vi "change_name.vi"(8 "error in (no error)":errorcluster, 9 "SerialNum":string, 10 "New Dev Name":string, 11 "Resources in":refnum<k20>[](array[refnum])) -> (0 "error out":errorcluster, 3 "Changed?":bool)   [LabVIEW 2015]
uses:
  <resource>/objmgr/nisysapi.rc
  <vilib>/nisyscfg/nisyscfg.lvlib
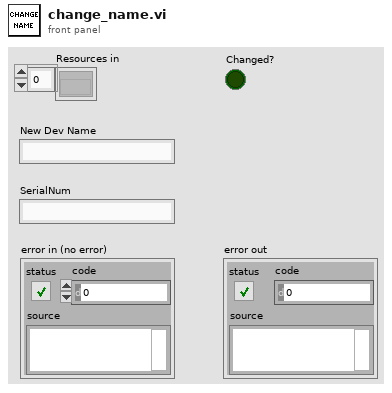
[diagram p1: front panel]
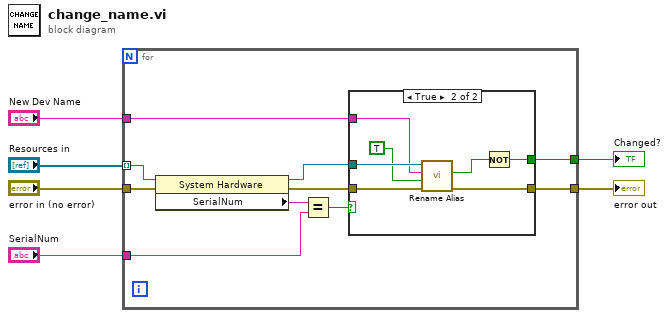
[diagram p0: block diagram]
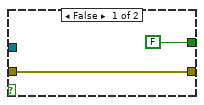
[diagram p2: hidden frame]
diagram:
  n1 = for {
    tunnel: "Resources in" -> [w16] mode=indexing
    tunnel: [w12] -> w4
    tunnel: "error in (no error)" -> [w15]
    tunnel: "New Dev Name" -> [w9]
    tunnel: "SerialNum" -> [w8]
    tunnel: [w7] -> w1
    n2 = property class="System Hardware"(reference=w16, error in=w15) -> (reference out=w14:refnum<k20>, error out=w13:errorcluster, "SerialNum"=w10:string)
    n3 = Equal?(x=w10, y=w8) -> (x = y?=w11:bool)
    n4 = case shown="True" w11 {
      tunnel: w14 -> [_ w25]
      tunnel: w13 -> [w18 w24]
      tunnel: [w18 w23] -> w12
      tunnel: w9 -> [_ w20]
      tunnel: [FALSE w19] -> w7
      frame False {
      }
      frame True {
        n5 = call <vilib>:"Rename Alias.vi"("error in (no error)"=w24, "Overwrite Conflict (F)"=TRUE ("overwrite (F)"), "New Name"=w20, "Resource in"=w25) -> ("error out"=w23:errorcluster, "Name Already Existed"=w21:bool)  [unwired: 4 in, 2 out]
        n6 = Not(x=w21) -> (.not. x?=w19:bool)
      }
    }
  }
  "error out" <- w4
  "Changed?" <- w1
